vi "Update.vi"(8 "error in (no error)":errorcluster, 10 "Text":string, 11 "Reverse Text in":refnum<class "Reverse Text.lvclass">) -> (0 "error out":errorcluster, 3 "Reverse Text out":refnum<class "Reverse Text.lvclass">)   [LabVIEW 2011, in "Reverse Text.lvclass"]
uses:
  Reverse Text.lvclass
  Reverse Text.lvclass/Reverse Text.ctl
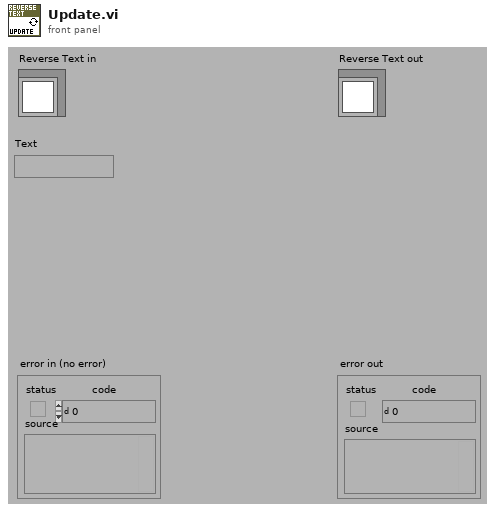
[diagram p1: front panel]
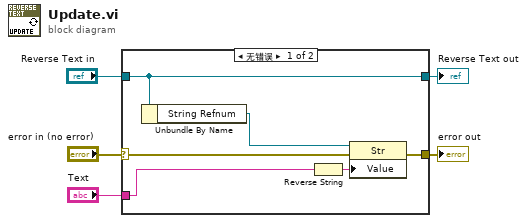
[diagram p0: block diagram]
diagram:
  n1 = case shown="无错误" "error in (no error)" {
    selector: "error in (no error)" -> [w8 w13]
    tunnel: "Reverse Text in" -> [w6 w12]
    tunnel: "Text" -> [w9 _]
    tunnel: [w7 w13] -> w2
    tunnel: [w6 w12] -> w1
    frame No Error {
      n2 = Unbundle By Name(w6) -> ("String Refnum"=w11:refnum<vi>)
      n3 = Reverse String(1:w9) -> (0:w10:string)
      n4 = property class="Str"(reference=w11, error in=w8, "Value"=w10) -> (error out=w7:errorcluster)  [unwired: 1 out]
    }
    frame Error {
    }
  }
  "Reverse Text out" <- w1
  "error out" <- w2
